vi "getImage.vi"(8 "error in (no error)":errorcluster, 10 "stop":bool, 11 "CameraAcquisitor in":refnum<class "CameraAcquisitor.lvclass">) -> (0 "error out":errorcluster, 2 "Array":path[](array[path]), 3 "CameraAcquisitor out":refnum<class "CameraAcquisitor.lvclass">)   [LabVIEW 2009, in "Hardware.lvlib" / "Channels.lvlib" / "CameraAcquisitor.lvclass"]
uses:
  CameraAcquisitor.lvclass
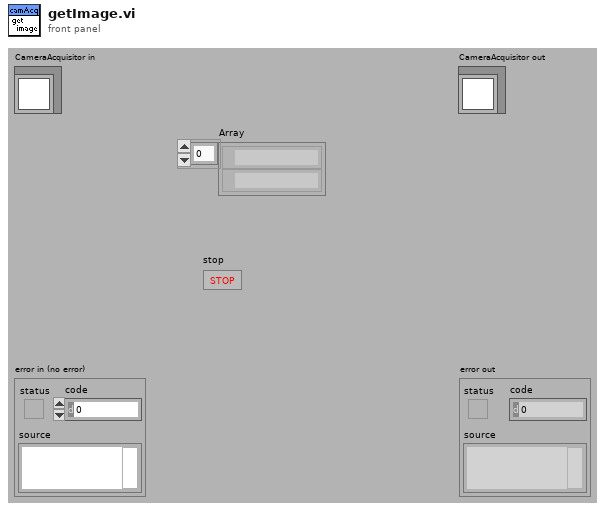
[diagram p1: front panel]
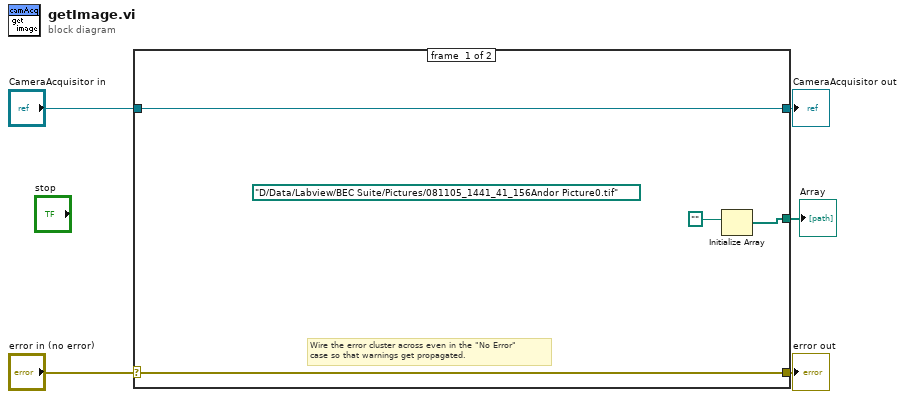
[diagram p0: block diagram]
diagram:
  n1 = case shown="No Error" "error in (no error)" {
    selector: "error in (no error)" -> [w8 w11]
    tunnel: [w8 w11] -> w4
    tunnel: [w9 w10] -> w2
    tunnel: "CameraAcquisitor in" -> [w9 w10]
    tunnel: [w7 _] -> w1
    frame #0 {
      (unwired) path "D:/Data/Labview/BEC Suite/Pictures/081105_1441_41_156Andor Picture0.tif"
      # "Wire the error cluster across even in the \"No Error\"\ncase so that warnings get propagated."
      n2 = Initialize Array(path "") -> (w7:path[])  [unwired: 1 in]
    }
    frame #1 {
    }
  }
  "error out" <- w4
  "CameraAcquisitor out" <- w2
  "Array" <- w1
